vi "calculate max turn.vi"(1 "parameters":T1={"max velocity (m/s)"=2.0, "wheel base width (m)"=0.7, "traverse CoF"=0.14}, 2 "Velocity (m/s)":dbl) -> (0 "max Ư":dbl)   [LabVIEW 2009]
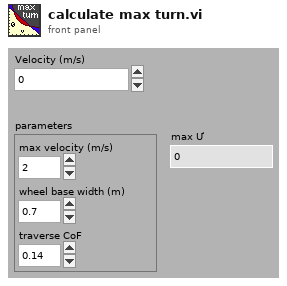
[diagram p1: front panel]
types:
  T1 = cluster{"max velocity (m/s)":dbl, "wheel base width (m)":dbl, "traverse CoF":dbl}
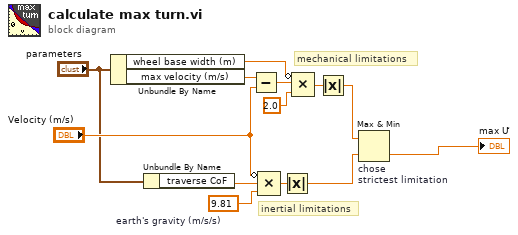
[diagram p0: block diagram]
diagram:
  w8 = 9.81  # earth's gravity (m/s/s)
  # "inertial limitations"
  # "mechanical limitations"
  n1 = Unbundle By Name("parameters") -> ("wheel base width (m)"=w6:dbl, "max velocity (m/s)"=w4:dbl)
  n2 = Unbundle By Name("parameters") -> ("traverse CoF"=w9:dbl)
  n3 = Subtract(x=w4, y="Velocity (m/s)") -> (x-y=w5:dbl)
  n4 = Compound Arithmetic op=MULTIPLY(invert "Velocity (m/s)", w9, w8) -> (w11:dbl)
  n5 = Absolute Value(x=w11) -> (abs(x)=w12:dbl)
  n6 = Compound Arithmetic op=MULTIPLY(invert w6, w5, 2.0 ("value")) -> (w10:dbl)
  n7 = Absolute Value(x=w10) -> (abs(x)=w13:dbl)
  n8 = Max & Min "chose\nstrictest limitation"(x=w13, y=w12) -> (min(x,y)=→"max Ư":dbl)  [unwired: 1 out]
